vi "Measure_Voltage.vi"(8 "error in (no error)":errorcluster, 10 "Measure_Configuration":variant, 11 "Function in":refnum<class "Function.lvclass">) -> (0 "error out":errorcluster, 2 "DC_Voltage":dbl[](array[numeric]), 3 "Function out":refnum<class "Function.lvclass">)   [LabVIEW 2020, in "Function.lvlib" / "Function.lvclass"]
uses:
  Function.lvclass
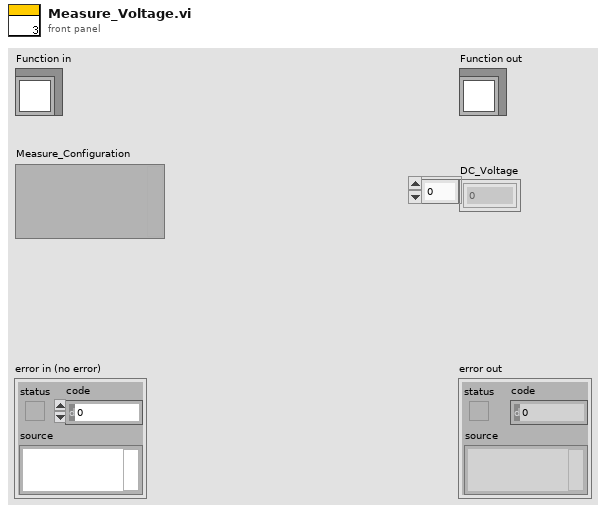
[diagram p1: front panel]
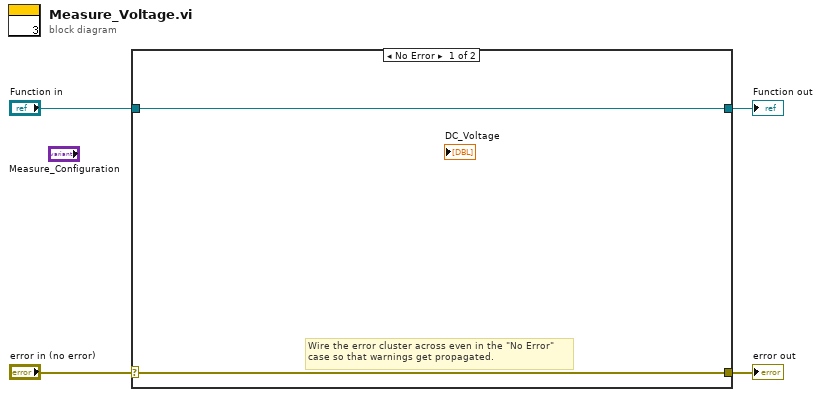
[diagram p0: block diagram]
diagram:
  n1 = case shown="No Error" "error in (no error)" {
    selector: "error in (no error)" -> [w5 w8]
    tunnel: [w5 w8] -> w3
    tunnel: [w6 w7] -> w1
    tunnel: "Function in" -> [w6 w7]
    frame No Error {
      # "Wire the error cluster across even in the \"No Error\"\ncase so that warnings get propagated."
    }
    frame Error {
    }
  }
  "error out" <- w3
  "Function out" <- w1
